vi "GetPlaylistListing.vi"(0 "Draw Area Size":T1) -> (1 "Cluster":T2, 2 "playlists":string[][](array[string]), 3 "Symbols":i32[](array[numeric]))   [LabVIEW 2014]
uses:
  <vilib>/Utility/miscctls.llb/LVBoundsTypeDef.ctl
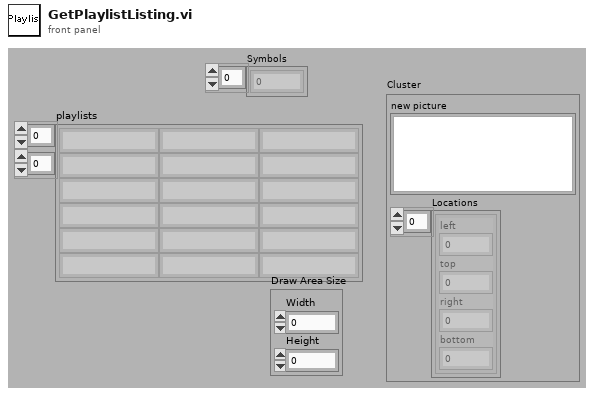
[diagram p1: front panel]
types:
  T1 = typedef "LVBoundsTypeDef.ctl" = cluster{"Width":u32, "Height":u32}
  T2 = cluster{"new picture":picture, "Locations":cluster{"left":i32, "top":i32, "right":i32, "bottom":i32}[]}
  T3 = cluster{"left":i32, "top":i32, "right":i32, "bottom":i32}[]
  T4 = cluster{"new picture out":picture, "Locations":cluster{"left":i32, "top":i32, "right":i32, "bottom":i32}[]}
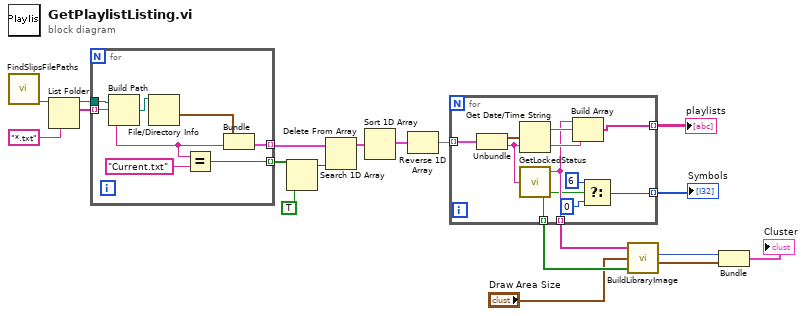
[diagram p0: block diagram]
diagram:
  n1 = call "FindSlipsFilePaths.vi"() -> ("Playlists"=w14:path)  [unwired: 2 in, 4 out]
  n2 = List Folder(path=w14, pattern="*.txt") -> (path out=w15:path, filenames=w16:string[])  [unwired: 2 in, 2 out]
  n3 = for {
    tunnel: w15 -> [w26]
    tunnel: w16 -> [w23] mode=indexing
    tunnel: [w24] -> w10 mode=indexing
    tunnel: [w21] -> w13 mode=indexing
    n4 = Build Path(base path=w26, name or relative path=w23) -> (appended path=w25:path)
    n5 = File/Directory Info(path=w25) -> (last mod=w20:timestamp)  [unwired: 1 in, 6 out]
    n6 = Equal?(x=w23, y="Current.txt") -> (x = y?=w21:bool)
    n7 = Bundle("last mod"=w20, w23) -> (w24:cluster{"last mod":timestamp, string})  [unwired: 1 in]
  }
  n8 = Search 1D Array(1D array=w13, element=TRUE) -> (index of element=w9:i32)  [unwired: 1 in]
  n9 = Delete From Array(array=w10, index=w9) -> (array with subset deleted=w11:cluster{"last mod":timestamp, string}[])  [unwired: 1 in, 1 out]
  n10 = Sort 1D Array(array=w11) -> (sorted array=w17:cluster{"last mod":timestamp, string}[])
  n11 = Reverse 1D Array(array=w17) -> (reversed array=w19:cluster{"last mod":timestamp, string}[])
  n12 = for {
    tunnel: w19 -> [w36] mode=indexing
    tunnel: [w35] -> w18 mode=indexing
    tunnel: [w31] -> w7 mode=indexing
    tunnel: [w28] -> w6 mode=indexing
    tunnel: [w27] -> w5 mode=indexing
    n13 = Unbundle(w36) -> ("last mod"=w34:timestamp, w32:string)
    n14 = Get Date/Time String(seconds (now)=w34) -> (date string=w33:string)  [unwired: 2 in, 1 out]
    n15 = call "GetLockedStatus.vi"("Filename"=w32) -> ("Locked?"=w27:bool, "Cleaned"=w28:string)  [unwired: 1 out]
    n16 = Build Array(w28, w33, w32) -> (w35:string[])
    n17 = Select(t=6, s=w27, f=0) -> (s? t:f=w31:i32)
  }
  "playlists" <- w18
  "Symbols" <- w7
  n18 = call "BuildLibraryImage.vi"("Array"=w5, "Draw Area Size"="Draw Area Size", "Books"=w6) -> ("Locations"=w3:T3, "new picture out"=w4:picture)
  n19 = Bundle("new picture out"=w4, "Locations"=w3) -> (→"Cluster":T4)  [unwired: 1 in]
